vi "udp sender.vi"   [LabVIEW 2012]
uses:
  <vilib>/Utility/tcp.llb/UDP Multicast Write-Only Open.vi
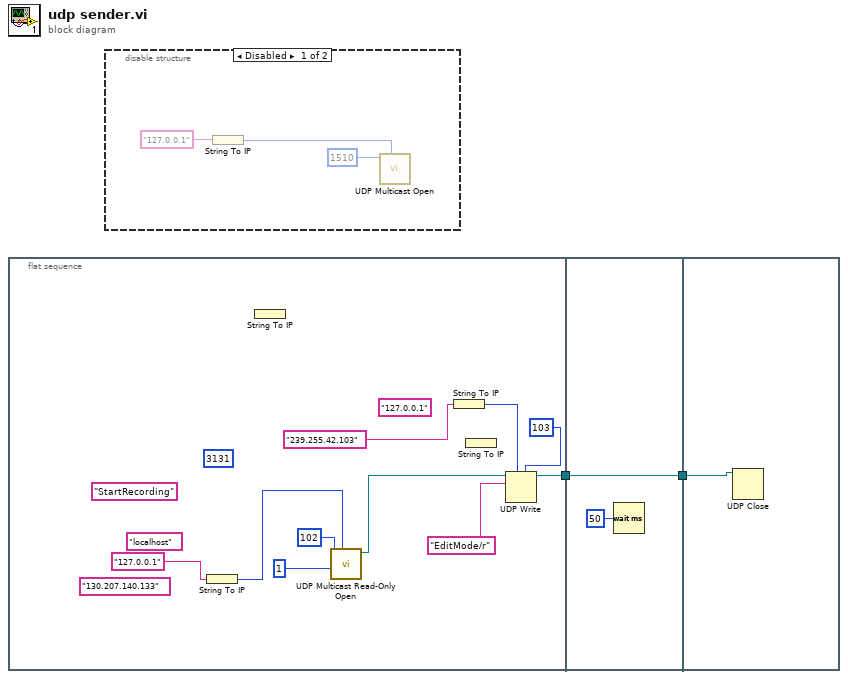
[diagram p0: block diagram]
diagram:
  n1 = flat-sequence {
    tunnel: [w11] -> w2
    tunnel: w2 -> [w14]
    tunnel: [w14] -> w1
    tunnel: w1 -> [w15]
    frame #0 {
      (unwired) "130.207.140.133" ("name")
      (unwired) "StartRecording" ("data in")
      (unwired) "127.0.0.1" ("name")
      (unwired) u16 3131 ("port")
      (unwired) "localhost" ("name")
      n2 = String To IP(1:"127.0.0.1" ("name")) -> (0:w9:u32)
      n3 = String To IP() -> ()  [unwired: 1 in, 1 out]
      n4 = call-poly "UDP Multicast Read-Only Open.vi"("net address"=w9, "time-to-live (1)"=u16 1, "port"=u16 102) -> ("connection ID"=w10:refnum<k16>)  [unwired: 2 in, 6 out]
      n5 = String To IP(1:"239.255.42.103" ("name")) -> (0:w7:u32)
      n6 = String To IP() -> ()  [unwired: 1 in, 1 out]
      n7 = UDP Write(address=w7, port or service name=u16 103 ("port"), connection ID=w10, data in="EditMode/r") -> (3:w11:refnum<k16>)  [unwired: 2 in, 1 out]
    }
    frame #1 {
      n8 = Wait (ms)(milliseconds to wait=u32 50) -> ()  [unwired: 1 out]
    }
    frame #2 {
      n9 = UDP Close(connection ID=w15) -> ()  [unwired: 1 in, 2 out]
    }
  }
  n10 = disable-structure shown="Disabled" {
    frame Disabled {
      n11 = String To IP(1:"127.0.0.1" ("name")) -> (0:w17:u32)
      n12 = call-poly <vilib>:"UDP Multicast Open.vi"("net address"=w17, "port"=u16 1510) -> ()  [unwired: 8 in, 2 out]
    }
    frame Enabled {
    }
  }
